vi "Untitled 10.vi"() -> ()   [LabVIEW 2017]
panel:
  out "Array":string[](array[string])
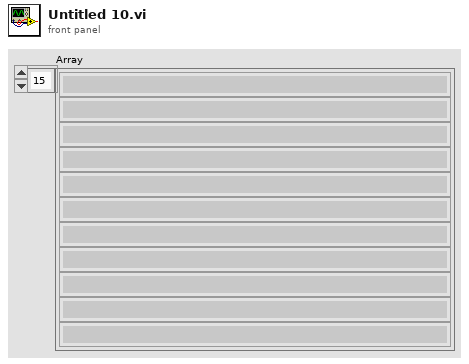
[diagram p1: front panel]
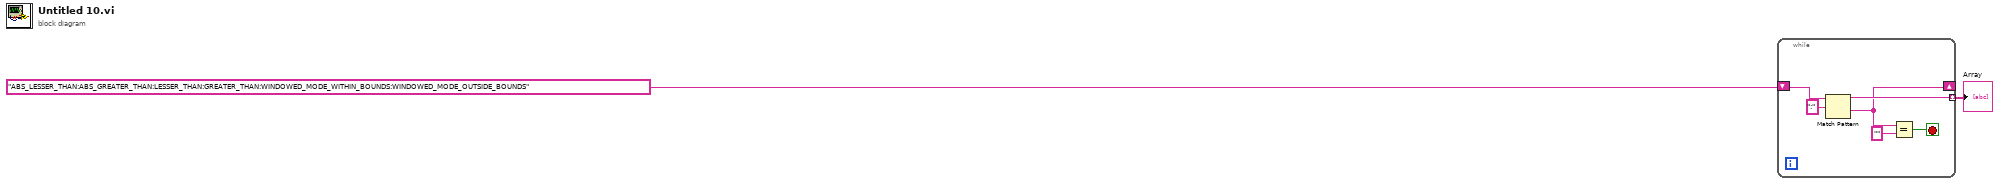
[diagram p0: block diagram]
diagram:
  n1 = while {
    shift-right: [w4] -> _
    shift-left: "ABS_LESSER_THAN:ABS_GREATER_THAN:LESSER_THAN:GREATER_THAN:WINDOWED_MODE_WITHIN_BOUNDS:WINDOWED_MODE_OUTSIDE_BOUNDS" -> [w8]
    tunnel: [w7] -> w1 mode=indexing
    stop <- w5 stop-if-true
    n2 = Match Pattern(string=w8, regular expression=":") -> (before substring=w7:string, after substring=w4:string)  [unwired: 1 in, 2 out]
    n3 = Equal?(x=w4, y="") -> (x = y?=w5:bool)
  }
  "Array" <- w1
